vi "Examen_03_Codigo.vi"() -> ()   [LabVIEW 2020]
uses:
  <vilib>/Instr/_visa.llb/VISA Configure Serial Port (Instr).vi
panel:
  in  "write buffer 3":string
  out "Temperatura 2":dbl
  in  "write buffer 2":string
  in  "Ingresar \nTemperatura":dbl
  in  "Modo manual":bool
  out "Temperatura DAQ":dbl
  in  "Stop Button":bool
  out "Numeric":i32
  in  "VISA resource name":refnum<visa-resource-name>
  # "APARADOR POR ESTACIONES"
  # "MODO AUTOMATICO"
  # "MODO MANUAL"
  # "TEMPERATURA REGISTRADA"
  # "INGRESA LA TEMPERATURA DESEADA"
  # "INVIERNO        <=10°"
  # "OTOÑO              10°>X >=18"
  # "TEMPERATURA REGISTRADA"
  # "PRIMAVERA  18°>X >=24°"
  # "PARA CAMBIAR A MODO MANUAL\nPRESIONAR EL SIGUIENTE BOTON"
  # "VERANO          > 24°"
  # "PUERTO COM"
  # "DATO ENVIADO"
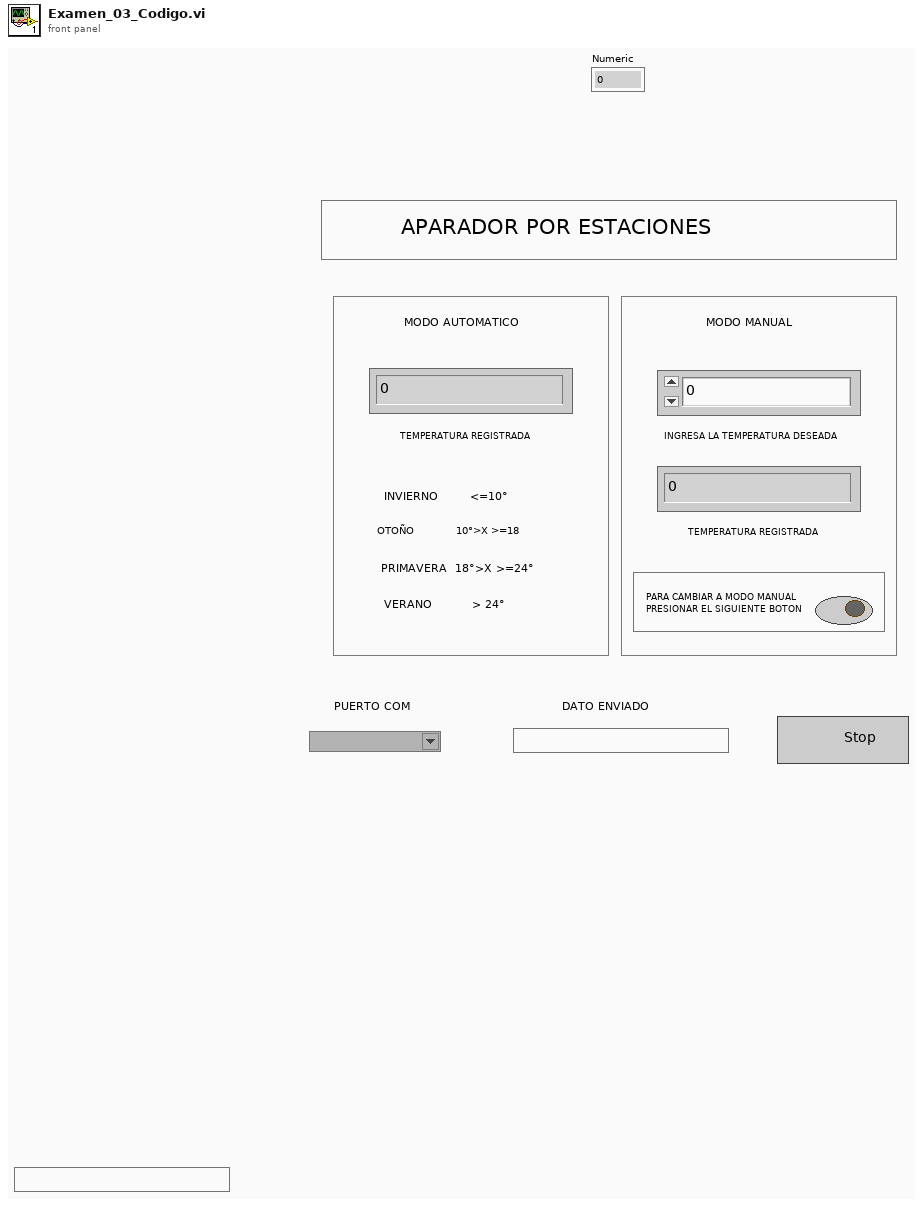
[diagram p1: front panel]
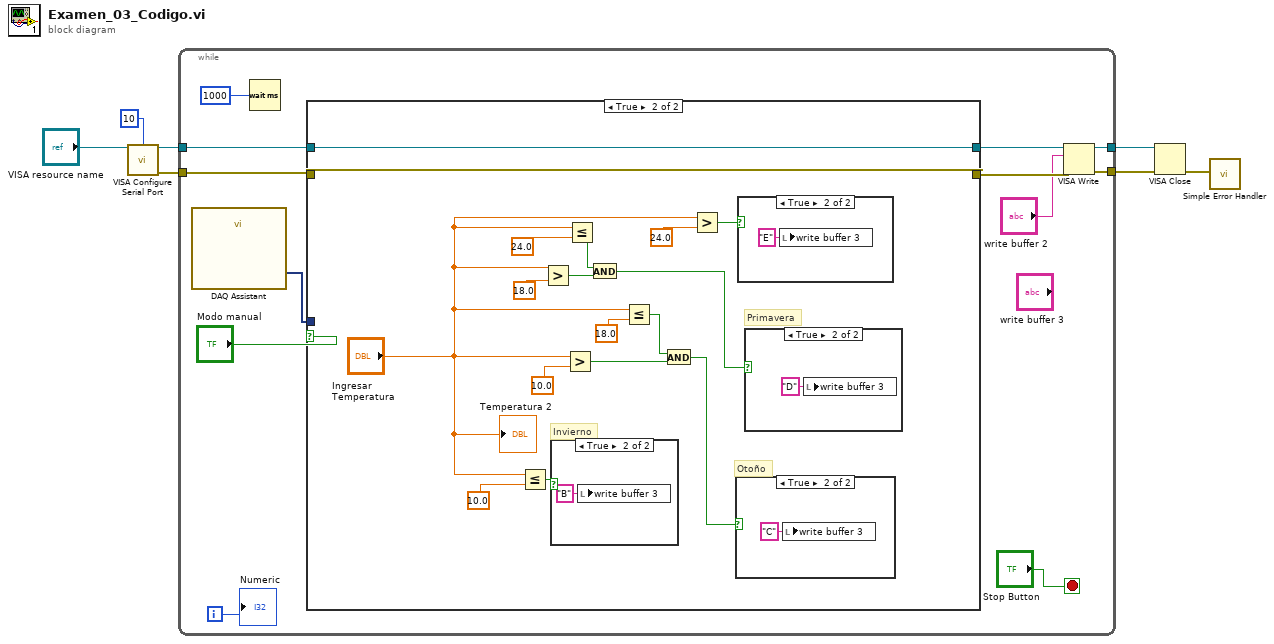
[diagram p0: block diagram]
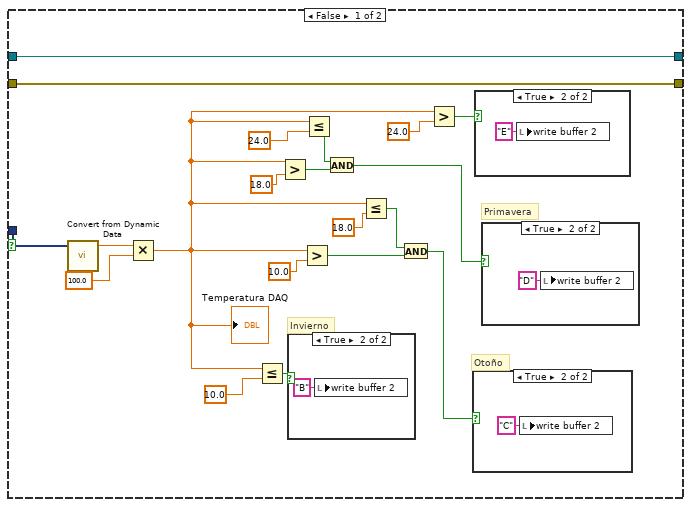
[diagram p2: hidden frame]
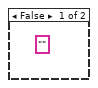
[diagram p6: hidden frame]
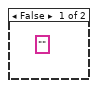
[diagram p10: hidden frame]
diagram:
  n1 = call-poly "VISA Configure Serial Port"("VISA resource name"="VISA resource name", "termination char\n(0xA = '\\n' = LF)"=u8 10 ("termination char\n(0xA = '\\n' = LF)")) -> ("VISA resource name out"=w5:refnum<visa-resource-name>, "error out"=w4:errorcluster)  [unwired: 12 in]
  n2 = while {
    tunnel: w5 -> [w14]
    tunnel: w4 -> [w13]
    tunnel: [w18] -> w2
    tunnel: [w17] -> w1
    i -> [w11]
    stop <- "Stop Button" stop-if-true
    n3 = call "DAQ Assistant"() -> ("data"=w8:dynamicdata)  [unwired: 17 in, 2 out]
    n4 = Wait (ms)(milliseconds to wait=u32 1000) -> ()  [unwired: 1 out]
    n5 = case shown="True" "Modo manual" {
      tunnel: w14 -> [w25 w60]
      tunnel: w13 -> [w24 w59]
      tunnel: [w25 w60] -> w16
      tunnel: [w24 w59] -> w15
      tunnel: w8 -> [w21 _]
      frame False {
        # "Primavera"
        # "Otoño"
        # "Invierno"
        n6 = call "Convert from Dynamic Data"("Dynamic Data Type"=w21) -> ("Scalar"=w23:dbl)  [unwired: 3 in]
        n7 = Multiply(x=w23, y=100.0) -> (x*y=w22:dbl)
        "Temperatura DAQ" <- w22
        n8 = Less Or Equal?(x=w22, y=10.0) -> (x <= y?=w37:bool)
        n9 = Greater?(x=w22, y=18.0) -> (0:w30:bool)
        n10 = case shown="True" w37 {
          frame False {
            (unwired) ""
          }
          frame True {
            n11 = local write "write buffer 2"("B" ("write buffer")) -> ()
          }
        }
        n12 = Greater?(x=w22, y=10.0) -> (0:w35:bool)
        n13 = Less Or Equal?(x=w22, y=24.0) -> (x <= y?=w31:bool)
        n14 = And(x=w31, y=w30) -> (x .and. y?=w28:bool)
        n15 = Less Or Equal?(x=w22, y=18.0) -> (x <= y?=w34:bool)
        n16 = And(x=w34, y=w35) -> (x .and. y?=w20:bool)
        n17 = Greater?(x=w22, y=24.0) -> (0:w26:bool)
        n18 = case shown="True" w20 {
          frame False {
          }
          frame True {
            n19 = local write "write buffer 2"("C" ("write buffer")) -> ()
          }
        }
        n20 = case shown="True" w26 {
          frame False {
          }
          frame True {
            n21 = local write "write buffer 2"("E" ("write buffer")) -> ()
          }
        }
        n22 = case shown="True" w28 {
          frame False {
          }
          frame True {
            n23 = local write "write buffer 2"("D" ("write buffer")) -> ()
          }
        }
      }
      frame True {
        # "Primavera"
        # "Otoño"
        # "Invierno"
        n24 = Less Or Equal?(x="Ingresar \nTemperatura", y=10.0) -> (x <= y?=w51:bool)
        n25 = Greater?(x="Ingresar \nTemperatura", y=18.0) -> (0:w55:bool)
        n26 = case shown="True" w51 {
          frame False {
            (unwired) ""
          }
          frame True {
            n27 = local write "write buffer 3"("B" ("write buffer")) -> ()
          }
        }
        n28 = Greater?(x="Ingresar \nTemperatura", y=10.0) -> (0:w52:bool)
        n29 = Less Or Equal?(x="Ingresar \nTemperatura", y=24.0) -> (x <= y?=w54:bool)
        n30 = And(x=w54, y=w55) -> (x .and. y?=w56:bool)
        n31 = Less Or Equal?(x="Ingresar \nTemperatura", y=18.0) -> (x <= y?=w53:bool)
        n32 = And(x=w53, y=w52) -> (x .and. y?=w58:bool)
        n33 = Greater?(x="Ingresar \nTemperatura", y=24.0) -> (0:w57:bool)
        n34 = case shown="True" w58 {
          frame False {
          }
          frame True {
            n35 = local write "write buffer 3"("C" ("write buffer")) -> ()
          }
        }
        n36 = case shown="True" w57 {
          frame False {
          }
          frame True {
            n37 = local write "write buffer 3"("E" ("write buffer")) -> ()
          }
        }
        n38 = case shown="True" w56 {
          frame False {
          }
          frame True {
            n39 = local write "write buffer 3"("D" ("write buffer")) -> ()
          }
        }
        "Temperatura 2" <- "Ingresar \nTemperatura"
      }
    }
    n40 = VISA Write(VISA resource name=w16, write buffer="write buffer 2", error in (no error)=w15) -> (VISA resource name out=w18:refnum<visa-resource-name>, error out=w17:errorcluster)  [unwired: 1 out]
    "Numeric" <- w11
  }
  n41 = VISA Close(VISA resource name=w2, error in (no error)=w1) -> (error out=w3:errorcluster)
  n42 = call <vilib>:"Simple Error Handler.vi"("error in (no error)"=w3) -> ()  [unwired: 4 in, 5 out]
